vi "Reset.vi"(8 "error in (no error)":errorcluster, 11 "VISA resource name":refnum<visa-resource-name>) -> (0 "error out":errorcluster, 3 "VISA resource name out":refnum<visa-resource-name>)   [LabVIEW 2016, in "Lake Shore 350.lvlib"]
doc: "Resets the instrument and then sends a set of default setup commands to the instrument."
uses:
  Lake Shore 350.lvlib
  Instance           1 13Saved   Reset .vi
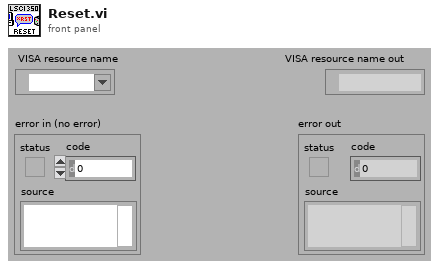
[diagram p1: front panel]
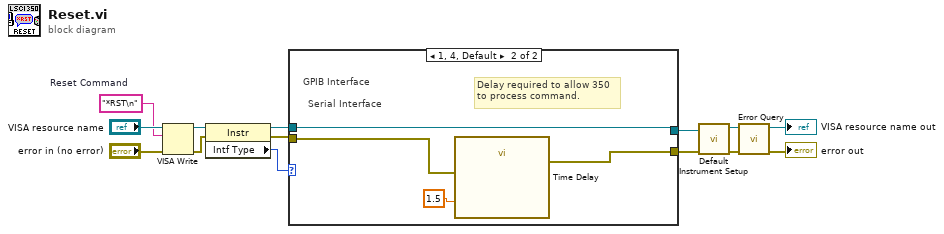
[diagram p0: block diagram]
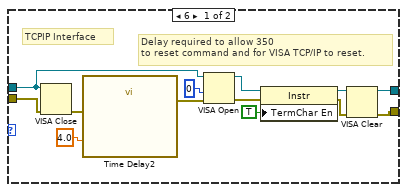
[diagram p2: hidden frame]
diagram:
  w12 = "*RST\n"  # Reset Command
  n1 = VISA Write(VISA resource name="VISA resource name", write buffer=w12, error in (no error)="error in (no error)") -> (VISA resource name out=w6:refnum<visa-resource-name>, error out=w5:errorcluster)  [unwired: 1 out]
  n2 = property class="Instr"(reference=w6, error in=w5) -> (reference out=w3:refnum<visa-resource-name>, error out=w4:errorcluster, "Intf Type"=w2:u16)
  n3 = case shown="1, 4, Default" w2 {
    tunnel: w4 -> [w27 w31]
    tunnel: [w17 w30] -> w7
    tunnel: w3 -> [w15 w28]
    tunnel: [w16 w28] -> w1
    frame 6 {
      # "Delay required to allow 350\nto reset command and for VISA TCP/IP to reset."
      # "TCPIP Interface"
      n4 = VISA Close(VISA resource name=w15, error in (no error)=w27) -> (error out=w25:errorcluster)
      n5 = call "Time Delay2"("error in (no error)"=w25, "Delay Time (s)"=4.0) -> ("error out"=w24:errorcluster)  [unwired: 9 in]
      n6 = VISA Open(access mode=u32 0, error in (no error)=w24, VISA resource name=w15) -> (VISA resource name=w19:refnum<visa-resource-name>, error out=w18:errorcluster)  [unwired: 2 in]
      n7 = property class="Instr"(reference=w19, error in=w18, "TermChar En"=TRUE) -> (reference out=w21:refnum<visa-resource-name>, error out=w20:errorcluster)
      n8 = VISA Clear(VISA resource name=w21, error in (no error)=w20) -> (VISA resource name out=w16:refnum<visa-resource-name>, error out=w17:errorcluster)
    }
    frame 1, 4, Default {
      # "Serial Interface"
      # "GPIB Interface"
      # "Delay required to allow 350\nto process command."
      n9 = call "Time Delay"("error in (no error)"=w31, "Delay Time (s)"=1.5) -> ("error out"=w30:errorcluster)  [unwired: 9 in]
    }
  }
  n10 = call "Default Instrument Setup.vi"("error in (no error)"=w7, "VISA resource name"=w1) -> ("error out"=w11:errorcluster, "VISA resource name out"=w10:refnum<visa-resource-name>)  [unwired: 8 in]
  n11 = call "Error Query.vi"("error in (no error)"=w11, "VISA resource name"=w10) -> ("error out"=→"error out":errorcluster, "VISA resource name out"=→"VISA resource name out":refnum<visa-resource-name>)  [unwired: 7 in, 1 out]
